vi "Harvest_Global.vi"() -> ()   [LabVIEW 2013]
panel:
  in  "stop":bool
  in  "Files Pulled 1":i32
  in  "Files Pulled 2":i32
  in  "Files pushed 1":i32
  in  "No Files to Pull":i32
  in  "Files pushed 2":i32
  in  "Done Transfer?":bool
  in  "No Files to Push":i32
  in  "File being transfered":path
  in  "Currently":string
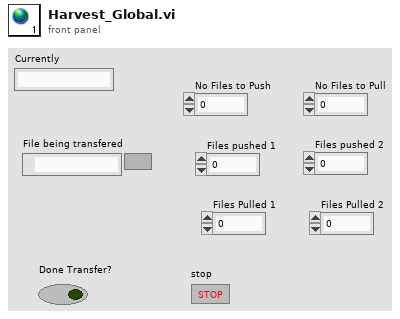
[diagram p1: front panel]
diagram:
